vi "Module Identities.vi"(8 "error in (no error)":errorcluster, 11 "Git Updater Module in":refnum<class "Git Updater Module.lvclass">) -> (0 "error out":errorcluster, 2 "Identities":refnum<class "Identity.lvclass">[](array[class]), 3 "Git Updater Module out":refnum<class "Git Updater Module.lvclass">)   [LabVIEW 2020, in "VolatusGUI.lvlib" / "Git Updater Module.lvclass"]
uses:
  Git Updater Module.lvclass
  Volatus/Identity/Identity.lvclass
  Config Updater Identity/Config Updater Identity.lvclass
  C:/dev/lv20CE/relink/lv-volatus/Volatus/Identity/Identity.lvclass
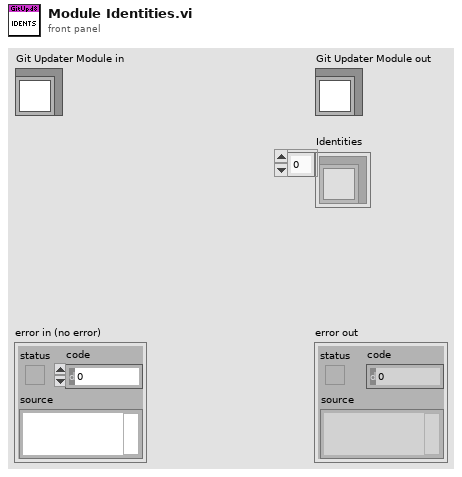
[diagram p1: front panel]
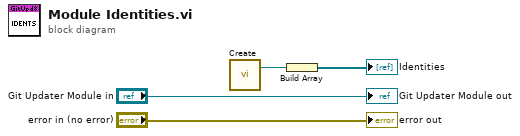
[diagram p0: block diagram]
diagram:
  n1 = call "Create.vi"() -> ("Config Updater Identity"=w2:refnum<class "Config Updater Identity.lvclass">)  [unwired: 7 in]
  n2 = Build Array(w2) -> (→"Identities":refnum<class "Config Updater Identity.lvclass">[])
  "error out" <- "error in (no error)"
  "Git Updater Module out" <- "Git Updater Module in"
